vi "1.vi"() -> ()   [LabVIEW 2016]
panel:
  out "Trace Position":dbl[](array[numeric])
  in  "Read Position":bool
  in  "Number of Seconds to Store":dbl=60.0
  in  "Apply X Scale":bool
  in  "Send Handshake":bool=TRUE
  out "DeviceIDs arranged by Type":u8[][](array[numeric])
  out "RoboRIO Net Address":u32
  out "Graph":cluster{sgl[], dbl[]}[](graph)
  in  "Update All Plots":bool
  in  "Reassign IP":bool
  in  "RoboRIO IP Address":string="10.27.67.2"
  in  "Plots":T1={"0"={"DeviceType"=2, "DeviceID"=0, "PropertyID"=1, "Current Value"=0.08333333333333333, "Y-Axis"=0, "Plot Color"=16777215, "Point Color"=16777216}, "0 2"={"DeviceType"=2, "DeviceID"=0, "PropertyID"=1, "Current Value"=50.0, "Y-Axis"=0, "Plot Color"=16777215, "Point Color"=16777216}, "0 3"={"DeviceType"=2, "DeviceID"=0, "PropertyID"=1, "Current Value"=50.0, "Y-Axis"=0, "Plot Color"=16777215, "Point Color"=16777216}, "0 4"={"DeviceType"=2, "DeviceID"=0, "PropertyID"=1, "Current Value"=50.0, "Y-Axis"=0, "Plot Color"=16777215, "Point Color"=16777216}, "0 5"={"DeviceType"=2, "DeviceID"=0, "PropertyID"=1, "Current Value"=50.0, "Y-Axis"=0, "Plot Color"=16777215, "Point Color"=16777216}, "0 6"={"DeviceType"=2, "DeviceID"=0, "PropertyID"=1, "Current Value"=50.0, "Y-Axis"=0, "Plot Color"=16777215, "Point Color"=16777216}, "0 7"={"DeviceType"=2, "DeviceID"=0, "PropertyID"=1, "Current Value"=50.0, "Y-Axis"=0, "Plot Color"=16777215, "Point Color"=16777216}, "0 8"={"DeviceType"=2, "DeviceID"=0, "PropertyID"=1, "Current Value"=50.0, "Y-Axis"=0, "Plot Color"=16777215, "Point Color"=16777216}, "0 9"={"DeviceType"=2, "DeviceID"=0, "PropertyID"=1, "Current Value"=50.0, "Y-Axis"=0, "Plot Color"=16777215, "Point Color"=16777216}, "0 10"={"DeviceType"=2, "DeviceID"=0, "PropertyID"=1, "Current Value"=50.0, "Y-Axis"=0, "Plot Color"=16777215, "Point Color"=16777216}, "0 11"={"DeviceType"=2, "DeviceID"=0, "PropertyID"=1, "Current Value"=50.0, "Y-Axis"=0, "Plot Color"=16777215, "Point Color"=16777216}, "0 12"={"DeviceType"=2, "DeviceID"=0, "PropertyID"=1, "Current Value"=50.0, "Y-Axis"=0, "Plot Color"=16777215, "Point Color"=16777216}, "0 13"={"DeviceType"=2, "DeviceID"=0, "PropertyID"=1, "Current Value"=50.0, "Y-Axis"=0, "Plot Color"=16777215, "Point Color"=16777216}, "0 14"={"DeviceType"=2, "DeviceID"=0, "PropertyID"=1, "Current Value"=50.0, "Y-Axis"=0, "Plot Color"=16777215, "Point Color"=16777216}, "0 15"={"DeviceType"=2, "DeviceID"=0, "PropertyID"=1, "Current Value"=50.0, "Y-Axis"=0, "Plot Color"=16777215, "Point Color"=16777216}, "0 16"={"DeviceType"=2, "DeviceID"=0, "PropertyID"=1, "Current Value"=50.0, "Y-Axis"=0, "Plot Color"=16777215, "Point Color"=16777216}} {"0 16"."DeviceID" items=["0"]; "0 16"."PropertyID" items=["PacketCounter", "Milliseconds Per Packet", "CPU Load"]; "0 16"."DeviceType" items=["Talon", "DIO", "RoboRIO"]; "0 16"."Y-Axis" items=["Red", "Green", "Blue", "Yellow"]; "0 15"."DeviceID" items=["0"]; "0 15"."PropertyID" items=["PacketCounter", "Milliseconds Per Packet", "CPU Load"]; "0 15"."DeviceType" items=["Talon", "DIO", "RoboRIO"]; "0 15"."Y-Axis" items=["Red", "Green", "Blue", "Yellow"]; "0 14"."DeviceID" items=["0"]; "0 14"."PropertyID" items=["PacketCounter", "Milliseconds Per Packet", "CPU Load"]; "0 14"."DeviceType" items=["Talon", "DIO", "RoboRIO"]; "0 14"."Y-Axis" items=["Red", "Green", "Blue", "Yellow"]; "0 13"."DeviceID" items=["0"]; "0 13"."PropertyID" items=["PacketCounter", "Milliseconds Per Packet", "CPU Load"]; "0 13"."DeviceType" items=["Talon", "DIO", "RoboRIO"]; "0 13"."Y-Axis" items=["Red", "Green", "Blue", "Yellow"]; "0 12"."DeviceID" items=["0"]; "0 12"."PropertyID" items=["PacketCounter", "Milliseconds Per Packet", "CPU Load"]; "0 12"."DeviceType" items=["Talon", "DIO", "RoboRIO"]; "0 12"."Y-Axis" items=["Red", "Green", "Blue", "Yellow"]; "0 11"."DeviceID" items=["0"]; "0 11"."PropertyID" items=["PacketCounter", "Milliseconds Per Packet", "CPU Load"]; "0 11"."DeviceType" items=["Talon", "DIO", "RoboRIO"]; "0 11"."Y-Axis" items=["Red", "Green", "Blue", "Yellow"]; "0 10"."DeviceID" items=["0"]; "0 10"."PropertyID" items=["PacketCounter", "Milliseconds Per Packet", "CPU Load"]; "0 10"."DeviceType" items=["Talon", "DIO", "RoboRIO"]; "0 10"."Y-Axis" items=["Red", "Green", "Blue", "Yellow"]; "0 9"."DeviceID" items=["0"]; "0 9"."PropertyID" items=["PacketCounter", "Milliseconds Per Packet", "CPU Load"]; "0 9"."DeviceType" items=["Talon", "DIO", "RoboRIO"]; "0 9"."Y-Axis" items=["Red", "Green", "Blue", "Yellow"]; "0 8"."DeviceID" items=["0"]; "0 8"."PropertyID" items=["PacketCounter", "Milliseconds Per Packet", "CPU Load"]; "0 8"."DeviceType" items=["Talon", "DIO", "RoboRIO"]; "0 8"."Y-Axis" items=["Red", "Green", "Blue", "Yellow"]; "0 7"."DeviceID" items=["0"]; "0 7"."PropertyID" items=["PacketCounter", "Milliseconds Per Packet", "CPU Load"]; "0 7"."DeviceType" items=["Talon", "DIO", "RoboRIO"]; "0 7"."Y-Axis" items=["Red", "Green", "Blue", "Yellow"]; "0 6"."DeviceID" items=["0"]; "0 6"."PropertyID" items=["PacketCounter", "Milliseconds Per Packet", "CPU Load"]; "0 6"."DeviceType" items=["Talon", "DIO", "RoboRIO"]; "0 6"."Y-Axis" items=["Red", "Green", "Blue", "Yellow"]; "0 5"."DeviceID" items=["0"]; "0 5"."PropertyID" items=["PacketCounter", "Milliseconds Per Packet", "CPU Load"]; "0 5"."DeviceType" items=["Talon", "DIO", "RoboRIO"]; "0 5"."Y-Axis" items=["Red", "Green", "Blue", "Yellow"]; "0 4"."DeviceID" items=["0"]; "0 4"."PropertyID" items=["PacketCounter", "Milliseconds Per Packet", "CPU Load"]; "0 4"."DeviceType" items=["Talon", "DIO", "RoboRIO"]; "0 4"."Y-Axis" items=["Red", "Green", "Blue", "Yellow"]; "0 3"."DeviceID" items=["0"]; "0 3"."PropertyID" items=["PacketCounter", "Milliseconds Per Packet", "CPU Load"]; "0 3"."DeviceType" items=["Talon", "DIO", "RoboRIO"]; "0 3"."Y-Axis" items=["Red", "Green", "Blue", "Yellow"]; "0 2"."DeviceID" items=["0"]; "0 2"."PropertyID" items=["PacketCounter", "Milliseconds Per Packet", "CPU Load"]; "0 2"."DeviceType" items=["Talon", "DIO", "RoboRIO"]; "0 2"."Y-Axis" items=["Red", "Green", "Blue", "Yellow"]; "0"."DeviceID" items=["0"]; "0"."PropertyID" items=["PacketCounter", "Milliseconds Per Packet", "CPU Load"]; "0"."DeviceType" items=["Talon", "DIO", "RoboRIO"]; "0"."Y-Axis" items=["Red", "Green", "Blue", "Yellow"]}
  in  "Load Config":bool
  in  "Save Config":bool
  in  "Configuation Path":path
  out "Real Milliseconds per Packet":sgl=50.0
  in  "Apply New Milliseconds":bool
  in  "Milliseconds per Packet":sgl=50.0
  in  "Number of Seconds Visible":dbl=10.0
  in  "Stop Data":bool
  # "Grapher v7.0"
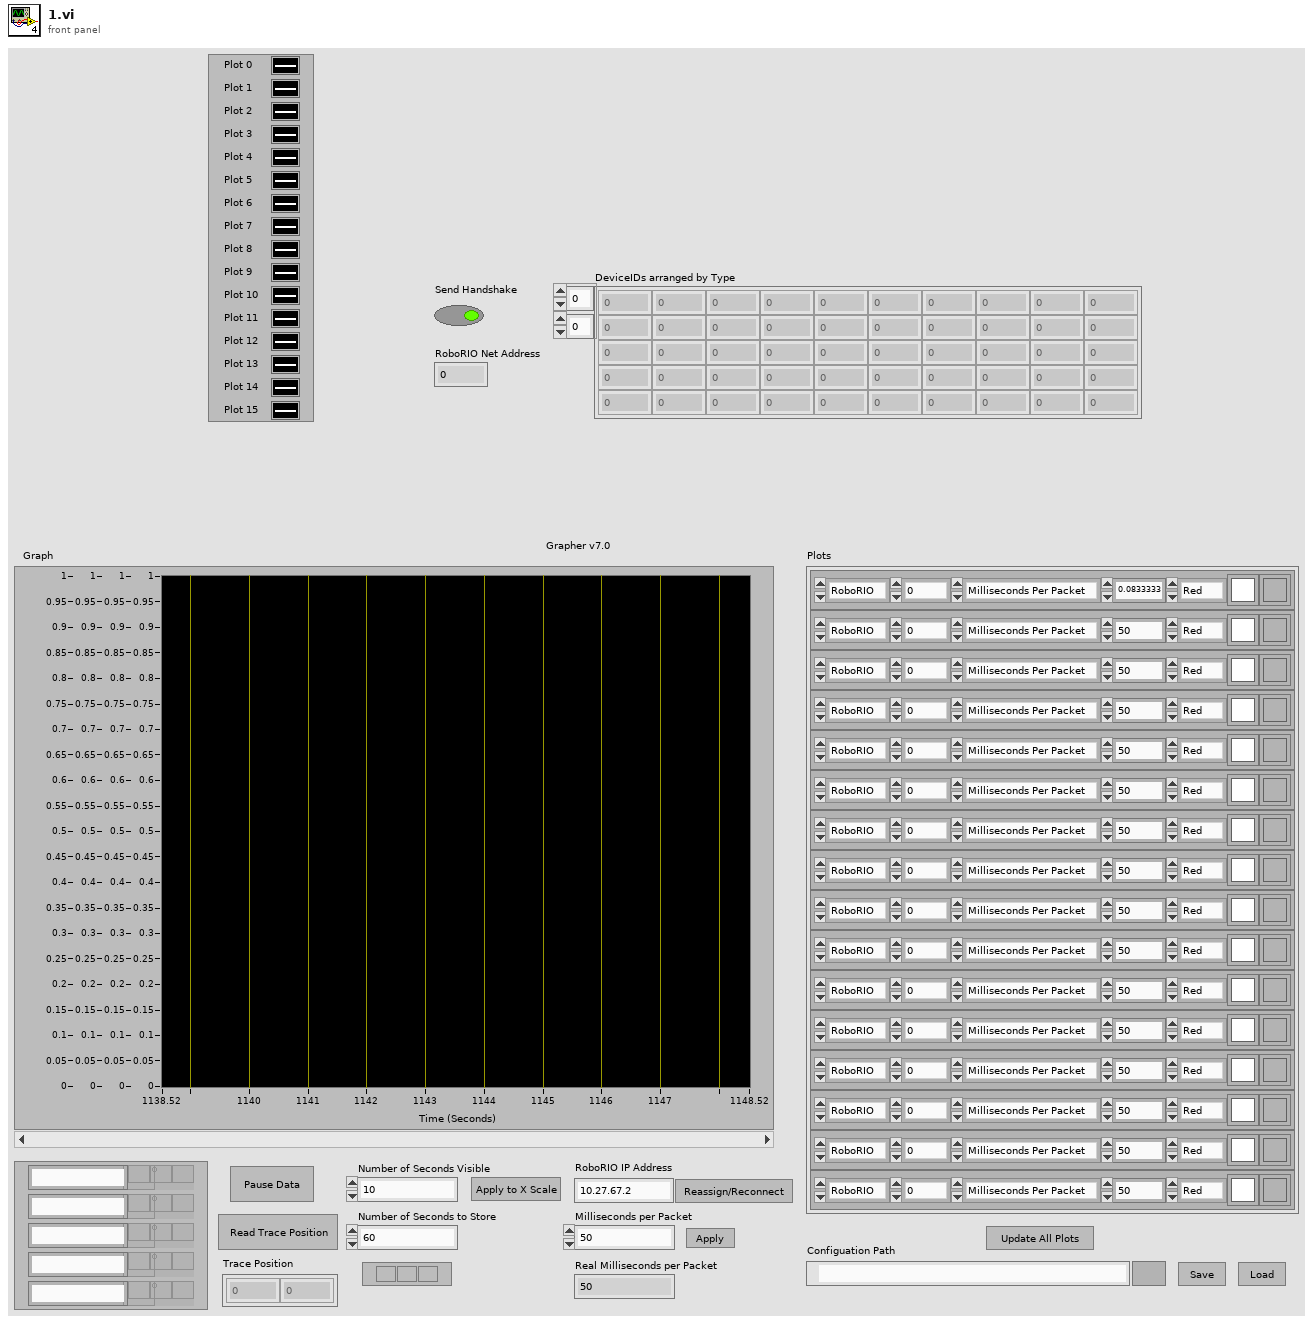
[diagram p1: front panel]
types:
  T1 = cluster{"0":cluster{"DeviceType":u8, "DeviceID":u8, "PropertyID":u8, "Current Value":dbl, "Y-Axis":u16, "Plot Color":u32, "Point Color":u32}, "0 2":cluster{"DeviceType":u8, "DeviceID":u8, "PropertyID":u8, "Current Value":dbl, "Y-Axis":u16, "Plot Color":u32, "Point Color":u32}, "0 3":cluster{"DeviceType":u8, "DeviceID":u8, "PropertyID":u8, "Current Value":dbl, "Y-Axis":u16, "Plot Color":u32, "Point Color":u32}, "0 4":cluster{"DeviceType":u8, "DeviceID":u8, "PropertyID":u8, "Current Value":dbl, "Y-Axis":u16, "Plot Color":u32, "Point Color":u32}, "0 5":cluster{"DeviceType":u8, "DeviceID":u8, "PropertyID":u8, "Current Value":dbl, "Y-Axis":u16, "Plot Color":u32, "Point Color":u32}, "0 6":cluster{"DeviceType":u8, "DeviceID":u8, "PropertyID":u8, "Current Value":dbl, "Y-Axis":u16, "Plot Color":u32, "Point Color":u32}, "0 7":cluster{"DeviceType":u8, "DeviceID":u8, "PropertyID":u8, "Current Value":dbl, "Y-Axis":u16, "Plot Color":u32, "Point Color":u32}, "0 8":cluster{"DeviceType":u8, "DeviceID":u8, "PropertyID":u8, "Current Value":dbl, "Y-Axis":u16, "Plot Color":u32, "Point Color":u32}, "0 9":cluster{"DeviceType":u8, "DeviceID":u8, "PropertyID":u8, "Current Value":dbl, "Y-Axis":u16, "Plot Color":u32, "Point Color":u32}, "0 10":cluster{"DeviceType":u8, "DeviceID":u8, "PropertyID":u8, "Current Value":dbl, "Y-Axis":u16, "Plot Color":u32, "Point Color":u32}, "0 11":cluster{"DeviceType":u8, "DeviceID":u8, "PropertyID":u8, "Current Value":dbl, "Y-Axis":u16, "Plot Color":u32, "Point Color":u32}, "0 12":cluster{"DeviceType":u8, "DeviceID":u8, "PropertyID":u8, "Current Value":dbl, "Y-Axis":u16, "Plot Color":u32, "Point Color":u32}, "0 13":cluster{"DeviceType":u8, "DeviceID":u8, "PropertyID":u8, "Current Value":dbl, "Y-Axis":u16, "Plot Color":u32, "Point Color":u32}, "0 14":cluster{"DeviceType":u8, "DeviceID":u8, "PropertyID":u8, "Current Value":dbl, "Y-Axis":u16, "Plot Color":u32, "Point Color":u32}, "0 15":cluster{"DeviceType":u8, "DeviceID":u8, "PropertyID":u8, "Current Value":dbl, "Y-Axis":u16, "Plot Color":u32, "Point Color":u32}, "0 16":cluster{"DeviceType":u8, "DeviceID":u8, "PropertyID":u8, "Current Value":dbl, "Y-Axis":u16, "Plot Color":u32, "Point Color":u32}}
  T2 = enum8{"DeviceListRequest", "DeviceList", "UpdateSubscription", "SubscriptionData"}
  T3 = enum8{"DeviceListRequest", "DeviceList", "UpdateSubscription", "SubscriptionData", "ChangeUpdateRate"}
  T4 = enum16{"open", "replace", "create", "open or create", "replace or create", "replace or create with confirmation"}
  T5 = cluster{"YScale.Maximum":dbl, "YScale.Minimum":dbl}
  T6 = typedef "LVAnnotationListTypeDef.ctl" = cluster{"Name":string, "Color":u32, "Style":u8, "Point Style":u8, "Name Visible":bool, "Allow Drag":bool, "Annotation Mode":u32, "Plot":i32, "Index":i32, "Position":cluster{"X":dbl, "Y":dbl}, "X Scale":u32, "Y Scale":u32, "Show Arrow":bool, "Lock Name":bool, "Plot Area":i32, "Label Offset":cluster{"X":dbl, "Y":dbl}}[]
  T7 = cluster{"Name":string, "Color":u32, "Style":u8, "Point Style":u8, "Name Visible":bool, "Allow Drag":bool, "Annotation Mode":u32, "Plot":i32, "Index":i32, "Position":cluster{"X":dbl, "Y":dbl}, "X Scale":u32, "Y Scale":u32, "Show Arrow":bool, "Lock Name":bool, "Plot Area":i32, "Label Offset":cluster{"X":dbl, "Y":dbl}}
  T8 = cluster{enum8{"DeviceListRequest", "DeviceList", "UpdateSubscription", "SubscriptionData"}, u8, "unsigned 8bit integer":u8, "unsigned 8bit integer":u8, "unsigned 8bit integer":u8}
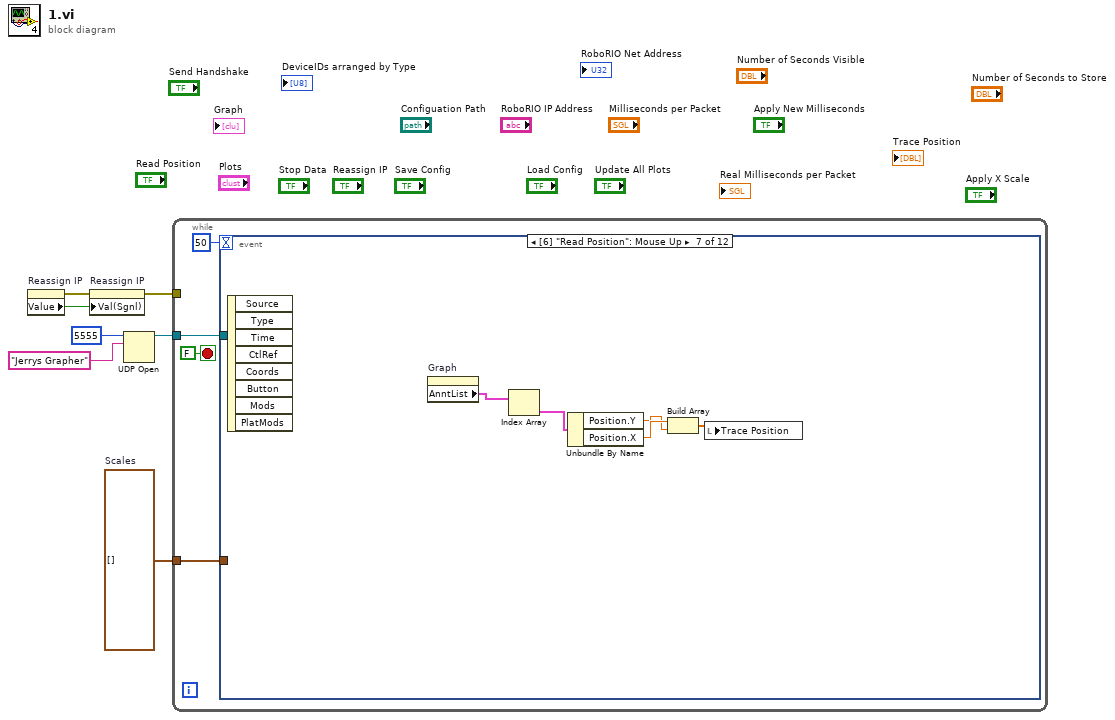
[diagram p0: block diagram]
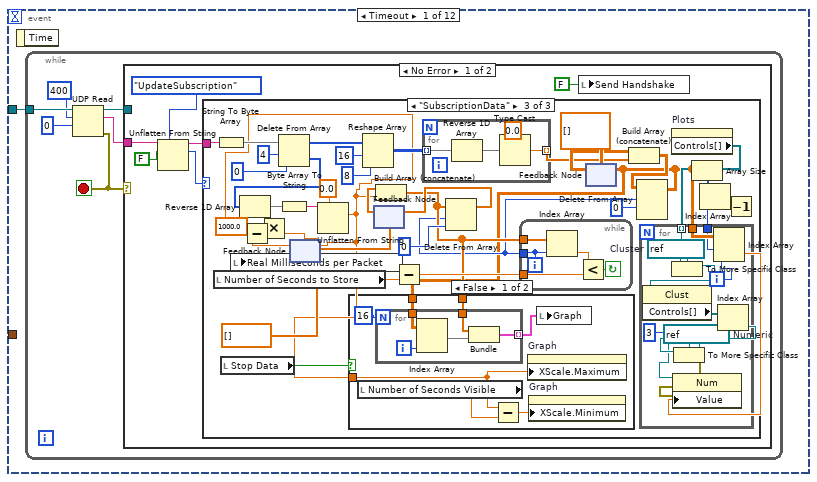
[diagram p2: hidden frame]
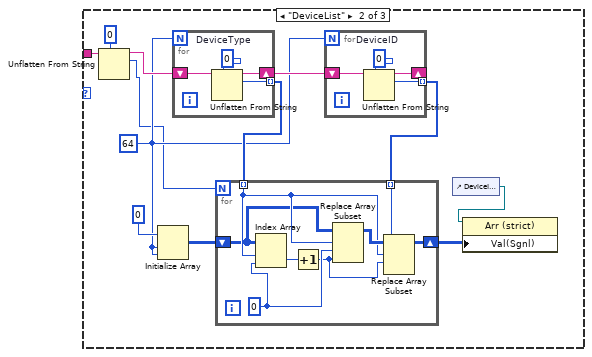
[diagram p4: hidden frame]
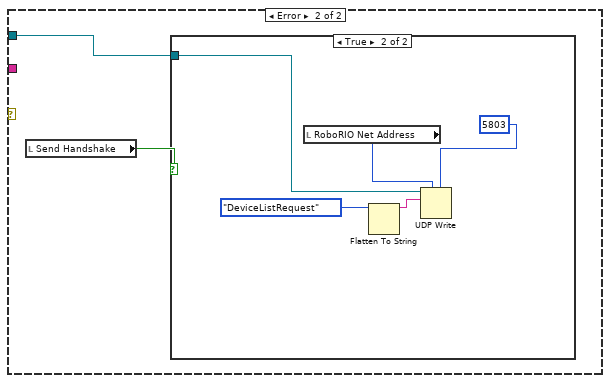
[diagram p6: hidden frame]
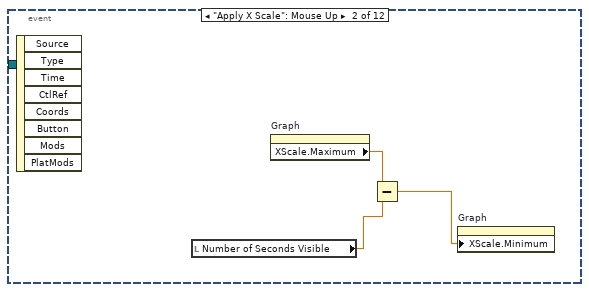
[diagram p8: hidden frame]
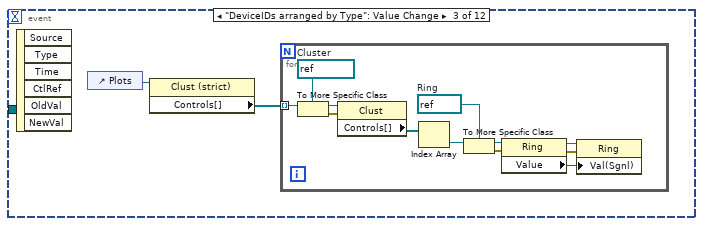
[diagram p9: hidden frame]
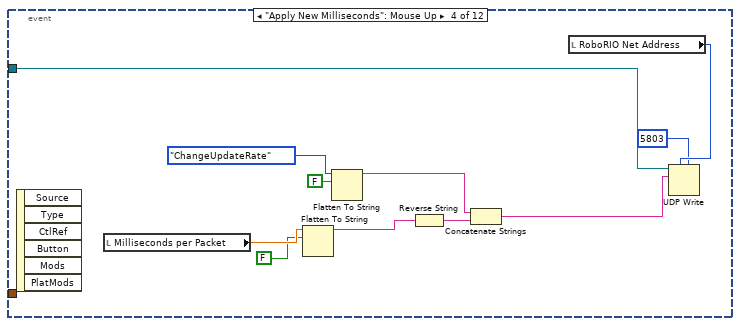
[diagram p10: hidden frame]
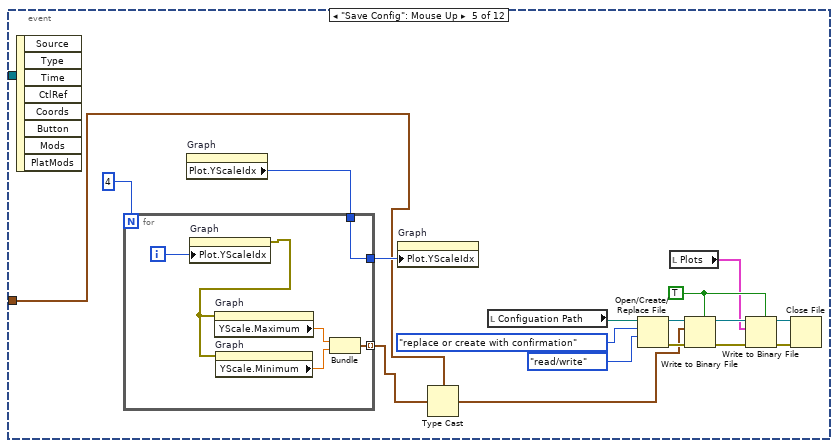
[diagram p11: hidden frame]
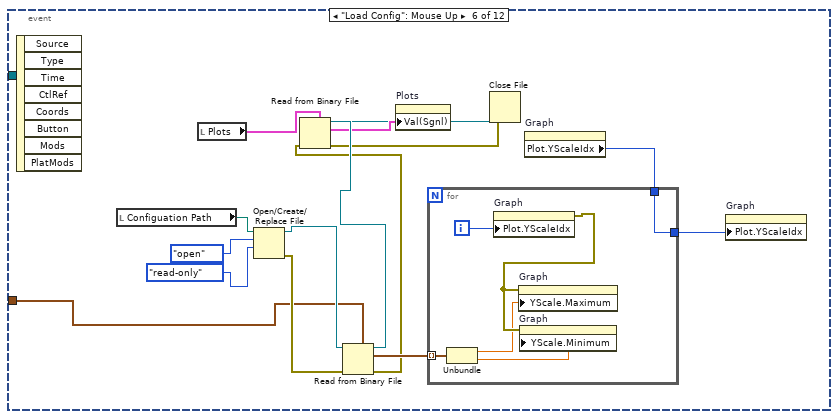
[diagram p12: hidden frame]
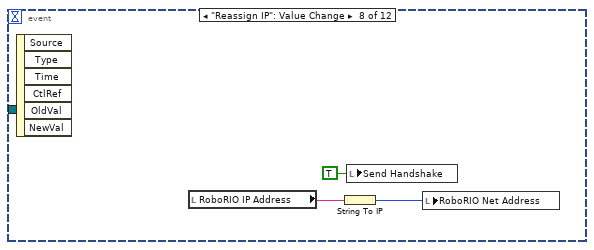
[diagram p13: hidden frame]
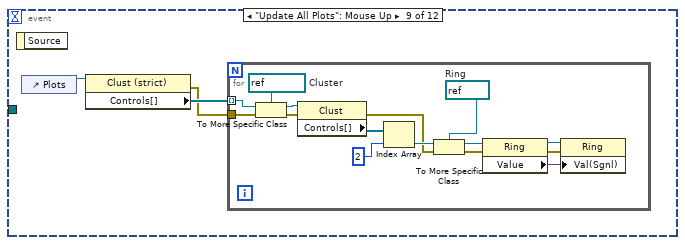
[diagram p14: hidden frame]
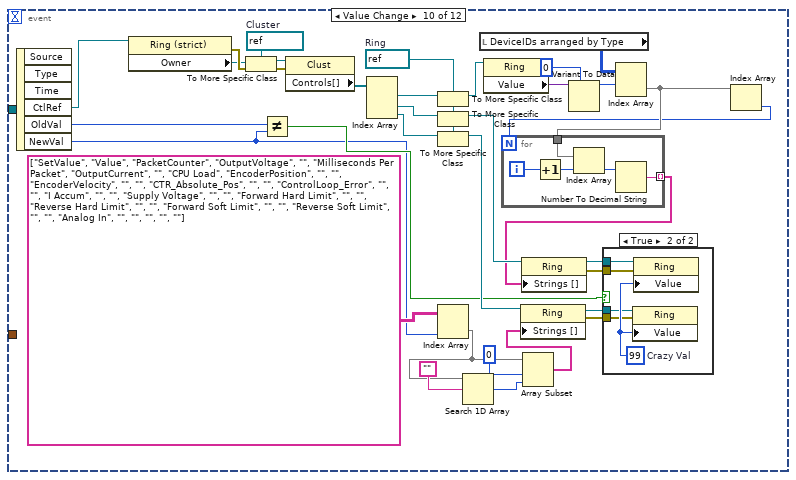
[diagram p15: hidden frame]
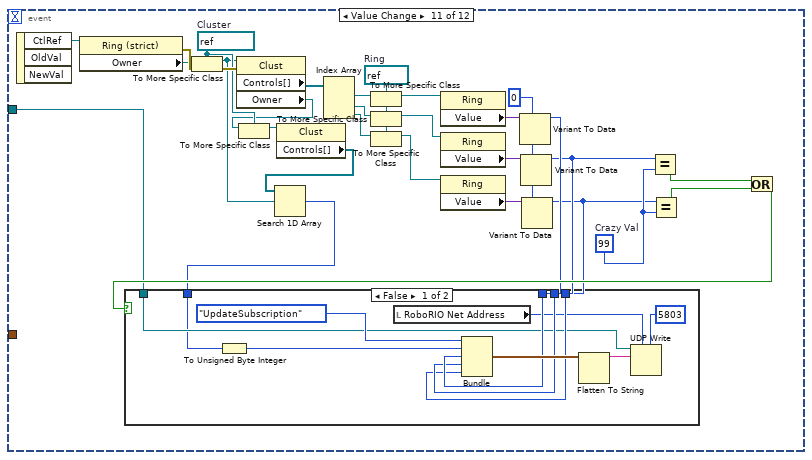
[diagram p17: hidden frame]
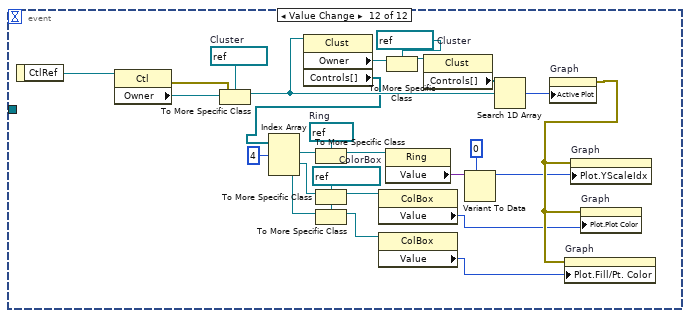
[diagram p19: hidden frame]
diagram:
  w1 = cluster{"Max":dbl, "Min":dbl}[] []  # Scales
  n1 = property on="Reassign IP" class="Bool (strict)"() -> (error out=w6:errorcluster, "Value"=w7:bool)  [unwired: 2 in, 1 out]
  n2 = property on="Reassign IP" class="Bool (strict)"(error in=w6, "Val(Sgnl)"=w7) -> (error out=w5:errorcluster)  [unwired: 1 in, 1 out]
  n3 = UDP Open(10:"Jerrys Grapher" ("service name"), 11:u16 5555 ("port")) -> (port=w4:refnum<k16>)  [unwired: 3 in, 2 out]
  n4 = while {
    tunnel: w5 -> [_]
    tunnel: w4 -> [w9]
    tunnel: w1 -> [w8]
    stop <- FALSE stop-if-true
    n5 = event shown="[6] \"Read Position\": Mouse Up" {
      selector: _ -> [_ _ _ _ _ _ _ _ _ _ _ _]
      dyn-events: _ -> [_ _ _ _ _ _ _ _ _ _ _ _]
      timeout: 50 -> [_ _ _ _ _ _ _ _ _ _ _ _]
      tunnel: w9 -> [w12 _ _ w149 _ _ _ _ _ _ w280 _]
      tunnel: w8 -> [_ _ _ _ w158 w181 _ _ _ _ _ _]
      event Timeout {
        n6 = event-data() -> ()  [unwired: 1 in, 1 out]
        n7 = while {
          tunnel: w12 -> [w18]
          stop <- w13 stop-if-true
          n8 = UDP Read(connection ID=w18, max size (548)=400 ("timeout ms (25000)"), timeout ms (25000)=0) -> (data out=w17:string, error out=w13:errorcluster, 3:w14:refnum<k16>)  [unwired: 1 in, 2 out]
          n9 = case shown="No Error" w13 {
            tunnel: w17 -> [w23 _]
            tunnel: w14 -> [_ w124]
            frame No Error {
              n10 = Unflatten From String(type=T2."UpdateSubscription", binary string=w23, data includes array or string size? (T)=FALSE) -> (rest of the binary string=w20:string, value=w21:T2)  [unwired: 2 in, 1 out]
              n11 = case shown="\"SubscriptionData\"" w21 {
                tunnel: w20 -> [_ w35 w85]
                frame "DeviceListRequest", Default {
                }
                frame "DeviceList" {
                  w26 = 64 ("JERRYSGRAPHER_MAX_NUMBER_OF_DEVICES")
                  n12 = Unflatten From String(type=u8 0 ("Number of Devices"), binary string=w35) -> (rest of the binary string=w34:string, value=w25:u8)  [unwired: 3 in, 1 out]
                  n13 = Initialize Array(u8 0, w26, w26) -> (w31:u8[][])
                  n14 = for {
                    N: w26 -> [_]
                    shift-right: [w49] -> w33
                    shift-left: w34 -> [w51]
                    tunnel: [w50] -> w30 mode=indexing
                    w52 = u8 0  # DeviceType
                    n15 = Unflatten From String(type=w52, binary string=w51) -> (rest of the binary string=w49:string, value=w50:u8)  [unwired: 3 in, 1 out]
                  }
                  n16 = for {
                    N: w26 -> [_]
                    shift-right: [w45] -> _
                    shift-left: w33 -> [w47]
                    tunnel: [w46] -> w29 mode=indexing
                    w48 = u8 0  # DeviceID
                    n17 = Unflatten From String(type=w48, binary string=w47) -> (rest of the binary string=w45:string, value=w46:u8)  [unwired: 3 in, 1 out]
                  }
                  n18 = for {
                    N: w25 -> [_]
                    tunnel: w30 -> [w42] mode=indexing
                    tunnel: w29 -> [w38] mode=indexing
                    shift-right: [w44] -> w28
                    shift-left: w31 -> [w40]
                    w41 = 0 ("disabled index (col)")
                    n19 = Index Array(array=w40, index (row)=w42, index (col)=w41) -> (element=w39:u8)
                    n20 = Increment(x=w39) -> (x+1=w37:u8)
                    n21 = Replace Array Subset(array=w40, new element=w37, index (row)=w42, index (col)=w41) -> (w43:u8[][])
                    n22 = Replace Array Subset(array=w43, new element=w38, index (row)=w42, index (col)=w37) -> (w44:u8[][])
                  }
                  n23 = control-ref of="DeviceIDs arranged by Type"() -> (w27:refnum<vi>)
                  n24 = property class="Arr (strict)"(reference=w27, "Val(Sgnl)"=w28) -> ()  [unwired: 1 in, 2 out]
                }
                frame "SubscriptionData" {
                  n25 = local read "Number of Seconds to Store"() -> (w70:dbl)
                  n26 = String To Byte Array(string=w85) -> (unsigned byte array=w86:u8[])
                  n27 = local read "Stop Data"() -> (w72:bool)
                  n28 = Delete From Array(array=w86, length=4, index=0) -> (deleted portion=w73:u8[], array with subset deleted=w80:u8[])
                  n29 = Reverse 1D Array(array=w73) -> (reversed array=w83:u8[])
                  n30 = Byte Array To String(unsigned byte array=w83) -> (string=w82:string)
                  n31 = feedback #1() -> (w56:sgl)  [unwired: 1 in]
                  n32 = Unflatten From String(type=sgl 0.0, binary string=w82) -> (value=w57:sgl)  [unwired: 3 in, 2 out]
                  n33 = Subtract(x=w57, y=w56) -> (x-y=w55:sgl)
                  n34 = Multiply(x=sgl 1000.0, y=w55) -> (x*y=w54:sgl)
                  n35 = local write "Real Milliseconds per Packet"(w54) -> ()
                  n36 = feedback-in #1(w57) -> ()
                  n37 = Reshape Array(w80, 16 ("dimension size"), 8 ("dimension size")) -> (w81:u8[][])
                  n38 = feedback #2(sgl[] []) -> (w77:sgl[])
                  n39 = Build Array (concatenate)(w77, w57) -> (w64:sgl[])
                  n40 = Subtract(x=w57, y=w70) -> (x-y=w69:dbl)
                  n41 = for {
                    tunnel: [w122] -> w74 mode=indexing
                    tunnel: w81 -> [w120] mode=indexing
                    n42 = Reverse 1D Array(array=w120) -> (reversed array=w119:u8[])
                    n43 = Type Cast(type=0.0, x=w119) -> (*(type *) &x=w122:dbl)
                  }
                  n44 = while {
                    tunnel: w69 -> [w104]
                    tunnel: w64 -> [w103]
                    tunnel: [w102] -> w63
                    i -> [w102]
                    stop <- w106 continue-if-true
                    n45 = Index Array(array=w103, index=w102) -> (element=w105:sgl)
                    n46 = Less?(x=w105, y=w104) -> (x < y?=w106:bool)
                  }
                  n47 = Delete From Array(array=w64, length=w63, index=0) -> (array with subset deleted=w67:sgl[])  [unwired: 1 out]
                  n48 = feedback-in #2(w67) -> ()
                  n49 = feedback #3(dbl[][] []) -> (w75:dbl[][])
                  n50 = Build Array (concatenate)(w75, w74) -> (w66:dbl[][])
                  n51 = Delete From Array(array=w66, length=w63, index (row)=0) -> (array with subset deleted=w61:dbl[][])  [unwired: 1 in, 1 out]
                  n52 = case shown="False" w72 {
                    tunnel: w57 -> [w113 _]
                    tunnel: w61 -> [w109 _]
                    tunnel: w64 -> [w108 _]
                    frame False {
                      n53 = local read "Number of Seconds Visible"() -> (w112:dbl)
                      n54 = for {
                        N: 16 -> [_]
                        tunnel: [w118] -> w107 mode=indexing
                        tunnel: w109 -> [w115]
                        tunnel: w108 -> [w114]
                        i -> [w117]
                        n55 = Index Array(array=w115, index (col)=w117) -> (element=w116:dbl[])  [unwired: 1 in]
                        n56 = Bundle(w114, w116) -> (w118:cluster{sgl[], dbl[]})  [unwired: 1 in]
                      }
                      n57 = Subtract(x=w113, y=w112) -> (x-y=w111:dbl)
                      n58 = property on="Graph" class="XYGraph (strict)"("XScale.Maximum"=w113) -> ()  [unwired: 2 in, 2 out]
                      n59 = property on="Graph" class="XYGraph (strict)"("XScale.Minimum"=w111) -> ()  [unwired: 2 in, 2 out]
                      n60 = local write "Graph"(w107) -> ()
                    }
                    frame True {
                    }
                  }
                  n61 = feedback-in #3(w61) -> ()
                  n62 = property on="Plots" class="Clust (strict)"() -> ("Controls[]"=w62:refnum<vi>[])  [unwired: 2 in, 2 out]
                  n63 = Array Size(array=w61) -> (size(s)=w60:i32[])
                  n64 = Index Array(array=w60) -> (element=w59:i32)  [unwired: 1 in]
                  n65 = Decrement(x=w59) -> (x-1=w58:i32)
                  n66 = for {
                    tunnel: w62 -> [w101] mode=indexing
                    tunnel: w61 -> [w92]
                    tunnel: w58 -> [w90]
                    i -> [w89]
                    w96 = refnum<vi> refnum  # Numeric
                    w100 = refnum<vi> refnum  # Cluster
                    n67 = To More Specific Class(target class=w100, reference=w101) -> (specific class reference=w99:refnum<vi>)  [unwired: 1 in, 1 out]
                    n68 = property class="Clust"(reference=w99) -> ("Controls[]"=w98:refnum<vi>[])  [unwired: 1 in, 2 out]
                    n69 = Index Array(array=w92, index (row)=w90, index (col)=w89) -> (element=w91:dbl)
                    n70 = Index Array(array=w98, index=3) -> (element=w95:refnum<vi>)
                    n71 = To More Specific Class(target class=w96, reference=w95) -> (specific class reference=w94:refnum<vi>, error out=w93:errorcluster)  [unwired: 1 in]
                    n72 = property class="Num"(reference=w94, error in=w93, "Value"=w91) -> ()  [unwired: 2 out]
                  }
                }
              }
              n73 = local write "Send Handshake"(FALSE ("Send Handshake")) -> ()
            }
            frame Error {
              n74 = local read "Send Handshake"() -> (w123:bool)
              n75 = case shown="True" w123 {
                tunnel: w124 -> [_ w127]
                frame False {
                }
                frame True {
                  n76 = local read "RoboRIO Net Address"() -> (w126:u32)
                  n77 = Flatten To String(anything=T2."DeviceListRequest") -> (data string=w128:string)  [unwired: 3 in, 2 out]
                  n78 = UDP Write(address=w126, port or service name=u16 5803 ("port"), connection ID=w127, data in=w128) -> ()  [unwired: 2 in, 2 out]
                }
              }
            }
          }
        }
      }
      event "Apply X Scale": Mouse Up {
        n79 = event-data() -> ()  [unwired: 1 in, 8 out]
        n80 = local read "Number of Seconds Visible"() -> (w131:dbl)
        n81 = property on="Graph" class="XYGraph (strict)"() -> ("XScale.Maximum"=w132:dbl)  [unwired: 2 in, 2 out]
        n82 = Subtract(x=w132, y=w131) -> (x-y=w130:dbl)
        n83 = property on="Graph" class="XYGraph (strict)"("XScale.Minimum"=w130) -> ()  [unwired: 2 in, 2 out]
      }
      event "DeviceIDs arranged by Type": Value Change {
        n84 = event-data() -> ()  [unwired: 1 in, 6 out]
        n85 = control-ref of="Plots"() -> (w134:refnum<vi>)
        n86 = property class="Clust (strict)"(reference=w134) -> ("Controls[]"=w133:refnum<vi>[])  [unwired: 1 in, 2 out]
        n87 = for {
          tunnel: w133 -> [w144] mode=indexing
          w140 = refnum<vi> refnum  # Ring
          w143 = refnum<vi> refnum  # Cluster
          n88 = To More Specific Class(target class=w143, reference=w144) -> (specific class reference=w145:refnum<vi>, error out=w146:errorcluster)  [unwired: 1 in]
          n89 = property class="Clust"(reference=w145, error in=w146) -> ("Controls[]"=w142:refnum<vi>[])  [unwired: 2 out]
          n90 = Index Array(array=w142) -> (element=w141:refnum<vi>)  [unwired: 1 in]
          n91 = To More Specific Class(target class=w140, reference=w141) -> (specific class reference=w139:refnum<vi>, error out=w138:errorcluster)  [unwired: 1 in]
          n92 = property class="Ring"(reference=w139, error in=w138) -> (reference out=w137:refnum<vi>, error out=w136:errorcluster, "Value"=w135:variant)
          n93 = property class="Ring"(reference=w137, error in=w136, "Val(Sgnl)"=w135) -> ()  [unwired: 2 out]
        }
      }
      event "Apply New Milliseconds": Mouse Up {
        n94 = event-data() -> ()  [unwired: 1 in, 6 out]
        n95 = local read "Milliseconds per Packet"() -> (w152:sgl)
        n96 = Flatten To String(anything=w152, prepend array or string size? (T)=FALSE) -> (data string=w154:string)  [unwired: 2 in, 2 out]
        n97 = Flatten To String(anything=T3."ChangeUpdateRate", prepend array or string size? (T)=FALSE) -> (data string=w153:string)  [unwired: 2 in, 2 out]
        n98 = Reverse String(1:w154) -> (0:w157:string)
        n99 = Concatenate Strings(w153, w157) -> (w156:string)
        n100 = local read "RoboRIO Net Address"() -> (w148:u32)
        n101 = UDP Write(address=w148, port or service name=u16 5803, connection ID=w149, data in=w156) -> ()  [unwired: 2 in, 2 out]
      }
      event "Save Config": Mouse Up {
        w171 = TRUE ("prepend array or string size? (T)")
        n102 = event-data() -> ()  [unwired: 1 in, 8 out]
        n103 = property on="Graph" class="XYGraph (strict)"() -> ("Plot.YScaleIdx"=w163:u32)  [unwired: 2 in, 2 out]
        n104 = for {
          N: 4 -> [_]
          tunnel: [w176] -> w164
          tunnel: w163 -> [w176]
          tunnel: [w175] -> w160 mode=indexing
          i -> [w180]
          n105 = property on="Graph" class="XYGraph (strict)"("Plot.YScaleIdx"=w180) -> (error out=w179:errorcluster)  [unwired: 2 in, 1 out]
          n106 = property on="Graph" class="XYGraph (strict)"(error in=w179) -> ("YScale.Maximum"=w178:dbl)  [unwired: 1 in, 2 out]
          n107 = property on="Graph" class="XYGraph (strict)"(error in=w179) -> ("YScale.Minimum"=w177:dbl)  [unwired: 1 in, 2 out]
          n108 = Bundle("YScale.Maximum"=w178, "YScale.Minimum"=w177) -> (w175:T5)  [unwired: 1 in]
        }
        n109 = property on="Graph" class="XYGraph (strict)"("Plot.YScaleIdx"=w164) -> ()  [unwired: 2 in, 2 out]
        n110 = Type Cast(type=w158, x=w160) -> (*(type *) &x=w159:cluster{"Max":dbl, "Min":dbl}[])
        n111 = local read "Configuation Path"() -> (w168:path)
        n112 = Open/Create/Replace File(file path (use dialog)=w168, operation (0:open)=T4."replace or create with confirmation", access (0:read/write)=enum16{"read/write", "read-only", "write-only"}."read/write") -> (refnum out=w170:refnum<file>, error out=w172:errorcluster)  [unwired: 3 in, 1 out]
        n113 = local read "Plots"() -> (w162:T1)
        n114 = Write to Binary File(file (use dialog)=w170, data=w159, error in=w172, 5:w171) -> (refnum out=w169:refnum<file>, error out=w173:errorcluster)  [unwired: 2 in, 1 out]
        n115 = Write to Binary File(file (use dialog)=w169, data=w162, error in=w173, 5:w171) -> (refnum out=w161:refnum<file>, error out=w174:errorcluster)  [unwired: 2 in, 1 out]
        n116 = Close File(refnum=w161, error in=w174) -> ()  [unwired: 2 out]
      }
      event "Load Config": Mouse Up {
        n117 = event-data() -> ()  [unwired: 1 in, 8 out]
        n118 = local read "Configuation Path"() -> (w195:path)
        n119 = local read "Plots"() -> (w187:T1)
        n120 = Open/Create/Replace File(file path (use dialog)=w195, operation (0:open)=T4."open", access (0:read/write)=enum16{"read/write", "read-only", "write-only"}."read-only") -> (refnum out=w192:refnum<file>, error out=w185:errorcluster)  [unwired: 3 in, 1 out]
        n121 = Read from Binary File(5:w181, 8:w185, 11:w192) -> (0:w184:errorcluster, 2:w189:cluster{"Max":dbl, "Min":dbl}[], 3:w188:refnum<file>)  [unwired: 3 in, 1 out]
        n122 = Read from Binary File(5:w187, 8:w184, 11:w188) -> (0:w183:errorcluster, 2:w186:T1, 3:w182:refnum<file>)  [unwired: 3 in, 1 out]
        n123 = property on="Plots" class="Clust (strict)"("Val(Sgnl)"=w186) -> ()  [unwired: 2 in, 2 out]
        n124 = Close File(refnum=w182, error in=w183) -> ()  [unwired: 2 out]
        n125 = property on="Graph" class="XYGraph (strict)"() -> ("Plot.YScaleIdx"=w191:u32)  [unwired: 2 in, 2 out]
        n126 = for {
          tunnel: [w199] -> w190
          tunnel: w191 -> [w199]
          tunnel: w189 -> [w198] mode=indexing
          i -> [w201]
          n127 = Unbundle(w198) -> ("Max"=w197:dbl, "Min"=w196:dbl)
          n128 = property on="Graph" class="XYGraph (strict)"("Plot.YScaleIdx"=w201) -> (error out=w200:errorcluster)  [unwired: 2 in, 1 out]
          n129 = property on="Graph" class="XYGraph (strict)"(error in=w200, "YScale.Maximum"=w197) -> ()  [unwired: 1 in, 2 out]
          n130 = property on="Graph" class="XYGraph (strict)"(error in=w200, "YScale.Minimum"=w196) -> ()  [unwired: 1 in, 2 out]
        }
        n131 = property on="Graph" class="XYGraph (strict)"("Plot.YScaleIdx"=w190) -> ()  [unwired: 2 in, 2 out]
      }
      event "Read Position": Mouse Up {
        n132 = event-data() -> ()  [unwired: 1 in, 8 out]
        n133 = property on="Graph" class="XYGraph (strict)"() -> ("AnntList"=w206:T6)  [unwired: 2 in, 2 out]
        n134 = Index Array(array=w206) -> (element=w205:T7)  [unwired: 1 in]
        n135 = Unbundle By Name(w205) -> ("Position.Y"=w203:dbl, "Position.X"=w204:dbl)
        n136 = Build Array(w204, w203) -> (w202:dbl[])
        n137 = local write "Trace Position"(w202) -> ()
      }
      event "Reassign IP": Value Change {
        n138 = event-data() -> ()  [unwired: 1 in, 6 out]
        n139 = local read "RoboRIO IP Address"() -> (w209:string)
        n140 = String To IP(1:w209) -> (0:w208:u32)
        n141 = local write "Send Handshake"(TRUE ("Send Handshake")) -> ()
        n142 = local write "RoboRIO Net Address"(w208) -> ()
      }
      event "Update All Plots": Mouse Up {
        n143 = event-data() -> ()  [unwired: 1 in, 1 out]
        n144 = control-ref of="Plots"() -> (w212:refnum<vi>)
        n145 = property class="Clust (strict)"(reference=w212) -> (error out=w210:errorcluster, "Controls[]"=w211:refnum<vi>[])  [unwired: 1 in, 1 out]
        n146 = for {
          tunnel: w211 -> [w226] mode=indexing
          tunnel: w210 -> [w223]
          w219 = refnum<vi> refnum  # Ring
          w227 = refnum<vi> refnum  # Cluster
          n147 = To More Specific Class(target class=w227, reference=w226, error in=w223) -> (specific class reference=w225:refnum<vi>, error out=w224:errorcluster)
          n148 = property class="Clust"(reference=w225, error in=w224) -> (error out=w216:errorcluster, "Controls[]"=w222:refnum<vi>[])  [unwired: 1 out]
          n149 = Index Array(array=w222, index=2) -> (element=w220:refnum<vi>)
          n150 = To More Specific Class(target class=w219, reference=w220, error in=w216) -> (specific class reference=w218:refnum<vi>, error out=w217:errorcluster)
          n151 = property class="Ring"(reference=w218, error in=w217) -> (reference out=w215:refnum<vi>, error out=w214:errorcluster, "Value"=w213:variant)
          n152 = property class="Ring"(reference=w215, error in=w214, "Val(Sgnl)"=w213) -> ()  [unwired: 2 out]
        }
      }
      event "Plots.0.DeviceType", "Plots.0 2.DeviceType", "Plots.0 3.DeviceType", "Plots.0 4.DeviceType", "Plots.0 5.DeviceType", "Plots.0 6.DeviceType", "Plots.0 7.DeviceType", "Plots.0 8.DeviceType", "Plots.0 9.DeviceType", "Plots.0 10.DeviceType", "Plots.0 11.DeviceType", "Plots.0 12.DeviceType", "Plots.0 13.DeviceType", "Plots.0 14.DeviceType", "Plots.0 15.DeviceType", "Plots.0 16.DeviceType": Value Change {
        w251 = refnum<vi> refnum  # Ring
        w256 = refnum<vi> refnum  # Cluster
        n153 = event-data() -> ("CtlRef"=w253:refnum<vi>, "OldVal"=w229:u8, "NewVal"=w228:u8)  [unwired: 1 in, 3 out]
        n154 = property class="Ring (strict)"(reference=w253) -> (error out=w255:errorcluster, "Owner"=w254:refnum<vi>)  [unwired: 1 in, 1 out]
        n155 = To More Specific Class(target class=w256, reference=w254, error in=w255) -> (specific class reference=w257:refnum<vi>, error out=w258:errorcluster)
        n156 = Not Equal?(x=w229, y=w228) -> (x != y?=w230:bool)
        n157 = property class="Clust"(reference=w257, error in=w258) -> ("Controls[]"=w259:refnum<vi>[])  [unwired: 2 out]
        n158 = Index Array(array=w259) -> (element #1=w260:refnum<vi>, element #2=w261:refnum<vi>, element #3=w252:refnum<vi>)  [unwired: 3 in]
        n159 = To More Specific Class(target class=w251, reference=w260) -> (specific class reference=w249:refnum<vi>)  [unwired: 1 in, 1 out]
        n160 = To More Specific Class(target class=w251, reference=w261) -> (specific class reference=w242:refnum<vi>)  [unwired: 1 in, 1 out]
        n161 = To More Specific Class(target class=w251, reference=w252) -> (specific class reference=w250:refnum<vi>)  [unwired: 1 in, 1 out]
        n162 = Index Array(array=string[][] [["SetValue", "Value", "PacketCounter"], ["OutputVoltage", "", "Milliseconds Per Packet"], ["OutputCurrent", "", "CPU Load"], ["EncoderPosition", "", ""], ["EncoderVelocity", "", ""], ["CTR_Absolute_Pos", "", ""], ["ControlLoop_Error", "", ""], ["I Accum", "", ""], ["Supply Voltage", "", ""], ["Forward Hard Limit", "", ""], ["Reverse Hard Limit", "", ""], ["Forward Soft Limit", "", ""], ["Reverse Soft Limit", "", ""], ["Analog In", "", ""], ["", "", ""]], index (col)=w228) -> (element=w237:string[])  [unwired: 1 in]
        n163 = Search 1D Array(1D array=w237, element="") -> (index of element=w238:i32)  [unwired: 1 in]
        n164 = local read "DeviceIDs arranged by Type"() -> (w246:u8[][])
        n165 = property class="Ring"(reference=w249) -> ("Value"=w248:variant)  [unwired: 1 in, 2 out]
        n166 = Array Subset(array=w237, index=0, length=w238) -> (w236:string[])
        n167 = property class="Ring"(reference=w250, "Strings []"=w236) -> (reference out=w232:refnum<vi>, error out=w231:errorcluster)  [unwired: 1 in]
        n168 = Variant To Data(type=u8 0 ("DeviceType"), Variant=w248) -> (data=w245:u8)  [unwired: 1 in, 1 out]
        n169 = Index Array(array=w246, index (row)=w245) -> (element=w244:u8[])  [unwired: 1 in]
        n170 = Index Array(array=w244) -> (element=w243:u8)  [unwired: 1 in]
        n171 = for {
          N: w243 -> [_]
          tunnel: w244 -> [w271]
          tunnel: [w267] -> w241 mode=indexing
          i -> [w270]
          n172 = Increment(x=w270) -> (x+1=w269:i32)
          n173 = Index Array(array=w271, index=w269) -> (element=w268:u8)
          n174 = Number To Decimal String(number=w268) -> (decimal integer string=w267:string)  [unwired: 1 in]
        }
        n175 = property class="Ring"(reference=w242, "Strings []"=w241) -> (reference out=w234:refnum<vi>, error out=w233:errorcluster)  [unwired: 1 in]
        n176 = case shown="True" w230 {
          tunnel: w234 -> [_ w266]
          tunnel: w233 -> [_ w265]
          tunnel: w232 -> [_ w263]
          tunnel: w231 -> [_ w262]
          frame False {
          }
          frame True {
            w264 = 99  # Crazy Val
            n177 = property class="Ring"(reference=w263, error in=w262, "Value"=w264) -> ()  [unwired: 2 out]
            n178 = property class="Ring"(reference=w266, error in=w265, "Value"=w264) -> ()  [unwired: 2 out]
          }
        }
      }
      event "Plots.0.DeviceID", "Plots.0.PropertyID", "Plots.0 2.DeviceID", "Plots.0 2.PropertyID", "Plots.0 3.DeviceID", "Plots.0 3.PropertyID", "Plots.0 4.DeviceID", "Plots.0 4.PropertyID", "Plots.0 5.DeviceID", "Plots.0 5.PropertyID", "Plots.0 6.DeviceID", "Plots.0 6.PropertyID", "Plots.0 7.DeviceID", "Plots.0 7.PropertyID", "Plots.0 8.DeviceID", "Plots.0 8.PropertyID", "Plots.0 9.DeviceID", "Plots.0 9.PropertyID", "Plots.0 10.DeviceID", "Plots.0 10.PropertyID", "Plots.0 11.DeviceID", "Plots.0 11.PropertyID", "Plots.0 12.DeviceID", "Plots.0 12.PropertyID", "Plots.0 13.DeviceID", "Plots.0 13.PropertyID", "Plots.0 14.DeviceID", "Plots.0 14.PropertyID", "Plots.0 15.DeviceID", "Plots.0 15.PropertyID", "Plots.0 16.DeviceID", "Plots.0 16.PropertyID": Value Change {
        w287 = 99  # Crazy Val
        w288 = u8 0 ("unsigned 8bit integer")
        w295 = refnum<vi> refnum  # Ring
        w277 = refnum<vi> refnum  # Cluster
        n179 = event-data() -> ("CtlRef"=w278:refnum<vi>)  [unwired: 1 in, 2 out]
        n180 = property class="Ring (strict)"(reference=w278) -> (error out=w298:errorcluster, "Owner"=w297:refnum<vi>)  [unwired: 1 in, 1 out]
        n181 = To More Specific Class(target class=w277, reference=w297, error in=w298) -> (specific class reference=w273:refnum<vi>, error out=w299:errorcluster)
        n182 = property class="Clust"(reference=w273, error in=w299) -> ("Controls[]"=w279:refnum<vi>[], "Owner"=w276:refnum<vi>)  [unwired: 2 out]
        n183 = To More Specific Class(target class=w277, reference=w276) -> (specific class reference=w275:refnum<vi>)  [unwired: 1 in, 1 out]
        n184 = property class="Clust"(reference=w275) -> ("Controls[]"=w274:refnum<vi>[])  [unwired: 1 in, 2 out]
        n185 = Search 1D Array(1D array=w274, element=w273) -> (index of element=w272:i32)  [unwired: 1 in]
        n186 = Index Array(array=w279) -> (element #1=w300:refnum<vi>, element #2=w301:refnum<vi>, element #3=w296:refnum<vi>)  [unwired: 3 in]
        n187 = To More Specific Class(target class=w295, reference=w300) -> (specific class reference=w294:refnum<vi>)  [unwired: 1 in, 1 out]
        n188 = To More Specific Class(target class=w295, reference=w301) -> (specific class reference=w293:refnum<vi>)  [unwired: 1 in, 1 out]
        n189 = To More Specific Class(target class=w295, reference=w296) -> (specific class reference=w292:refnum<vi>)  [unwired: 1 in, 1 out]
        n190 = property class="Ring"(reference=w294) -> ("Value"=w289:variant)  [unwired: 1 in, 2 out]
        n191 = property class="Ring"(reference=w293) -> ("Value"=w290:variant)  [unwired: 1 in, 2 out]
        n192 = property class="Ring"(reference=w292) -> ("Value"=w291:variant)  [unwired: 1 in, 2 out]
        n193 = Variant To Data(type=w288, Variant=w289) -> (data=w283:u8)  [unwired: 1 in, 1 out]
        n194 = Variant To Data(type=w288, Variant=w290) -> (data=w282:u8)  [unwired: 1 in, 1 out]
        n195 = Variant To Data(type=w288, Variant=w291) -> (data=w281:u8)  [unwired: 1 in, 1 out]
        n196 = Equal?(x=w282, y=w287) -> (x = y?=w285:bool)
        n197 = Equal?(x=w281, y=w287) -> (x = y?=w286:bool)
        n198 = Or(x=w285, y=w286) -> (x .or. y?=w284:bool)
        n199 = case shown="False" w284 {
          tunnel: w283 -> [w308 _]
          tunnel: w282 -> [w307 _]
          tunnel: w281 -> [w306 _]
          tunnel: w280 -> [w305 _]
          tunnel: w272 -> [w302 _]
          frame False {
            n200 = To Unsigned Byte Integer(number=w302) -> (unsigned 8bit integer=w309:u8)
            n201 = local read "RoboRIO Net Address"() -> (w304:u32)
            n202 = Bundle(T2."UpdateSubscription", w309, "unsigned 8bit integer"=w308, "unsigned 8bit integer"=w307, "unsigned 8bit integer"=w306) -> (w311:T8)  [unwired: 1 in]
            n203 = Flatten To String(anything=w311) -> (data string=w312:string)  [unwired: 3 in, 2 out]
            n204 = UDP Write(address=w304, port or service name=u16 5803, connection ID=w305, data in=w312) -> ()  [unwired: 2 in, 2 out]
          }
          frame True {
          }
        }
      }
      event "Plots.0.Y-Axis", "Plots.0 2.Y-Axis", "Plots.0 3.Y-Axis", "Plots.0 4.Y-Axis", "Plots.0 5.Y-Axis", "Plots.0 6.Y-Axis", "Plots.0 7.Y-Axis", "Plots.0 8.Y-Axis", "Plots.0 9.Y-Axis", "Plots.0 10.Y-Axis", "Plots.0 11.Y-Axis", "Plots.0 12.Y-Axis", "Plots.0 13.Y-Axis", "Plots.0 14.Y-Axis", "Plots.0 15.Y-Axis", "Plots.0 16.Y-Axis", "Plots.0.Plot Color", "Plots.0 2.Plot Color", "Plots.0 3.Plot Color", "Plots.0 4.Plot Color", "Plots.0 5.Plot Color", "Plots.0 6.Plot Color", "Plots.0 7.Plot Color", "Plots.0 8.Plot Color", "Plots.0 9.Plot Color", "Plots.0 10.Plot Color", "Plots.0 11.Plot Color", "Plots.0 12.Plot Color", "Plots.0 13.Plot Color", "Plots.0 14.Plot Color", "Plots.0 15.Plot Color", "Plots.0 16.Plot Color", "Plots.0.Point Color", "Plots.0 2.Point Color", "Plots.0 3.Point Color", "Plots.0 4.Point Color", "Plots.0 5.Point Color", "Plots.0 6.Point Color", "Plots.0 7.Point Color", "Plots.0 8.Point Color", "Plots.0 9.Point Color", "Plots.0 10.Point Color", "Plots.0 11.Point Color", "Plots.0 12.Point Color", "Plots.0 13.Point Color", "Plots.0 14.Point Color", "Plots.0 15.Point Color", "Plots.0 16.Point Color": Value Change {
        w317 = refnum<vi> refnum  # ColorBox
        w328 = refnum<vi> refnum  # Ring
        w331 = refnum<vi> refnum  # Cluster
        w336 = refnum<vi> refnum  # Cluster
        n205 = event-data() -> ("CtlRef"=w335:refnum<vi>)  [unwired: 1 in]
        n206 = property class="Ctl"(reference=w335) -> (error out=w338:errorcluster, "Owner"=w337:refnum<vi>)  [unwired: 1 in, 1 out]
        n207 = To More Specific Class(target class=w336, reference=w337, error in=w338) -> (specific class reference=w333:refnum<vi>)  [unwired: 1 out]
        n208 = property class="Clust"(reference=w333) -> ("Owner"=w332:refnum<vi>, "Controls[]"=w319:refnum<vi>[])  [unwired: 1 in, 2 out]
        n209 = Index Array(array=w319, index #1=4 ("index")) -> (element #1=w322:refnum<vi>, element #2=w321:refnum<vi>, element #3=w320:refnum<vi>)  [unwired: 2 in]
        n210 = To More Specific Class(target class=w328, reference=w322) -> (specific class reference=w327:refnum<vi>)  [unwired: 1 in, 1 out]
        n211 = To More Specific Class(target class=w317, reference=w321) -> (specific class reference=w326:refnum<vi>)  [unwired: 1 in, 1 out]
        n212 = To More Specific Class(target class=w317, reference=w320) -> (specific class reference=w325:refnum<vi>)  [unwired: 1 in, 1 out]
        n213 = property class="ColBox"(reference=w326) -> ("Value"=w314:u32)  [unwired: 1 in, 2 out]
        n214 = property class="ColBox"(reference=w325) -> ("Value"=w313:u32)  [unwired: 1 in, 2 out]
        n215 = property class="Ring"(reference=w327) -> ("Value"=w324:variant)  [unwired: 1 in, 2 out]
        n216 = To More Specific Class(target class=w331, reference=w332) -> (specific class reference=w330:refnum<vi>)  [unwired: 1 in, 1 out]
        n217 = property class="Clust"(reference=w330) -> ("Controls[]"=w329:refnum<vi>[])  [unwired: 1 in, 2 out]
        n218 = Variant To Data(type=u8 0 ("unsigned 8bit integer"), Variant=w324) -> (data=w315:u8)  [unwired: 1 in, 1 out]
        n219 = Search 1D Array(1D array=w329, element=w333) -> (index of element=w334:i32)  [unwired: 1 in]
        n220 = property on="Graph" class="XYGraph (strict)"("Active Plot"=w334) -> (error out=w316:errorcluster)  [unwired: 2 in, 1 out]
        n221 = property on="Graph" class="XYGraph (strict)"(error in=w316, "Plot.Fill/Pt. Color"=w313) -> ()  [unwired: 1 in, 2 out]
        n222 = property on="Graph" class="XYGraph (strict)"(error in=w316, "Plot.YScaleIdx"=w315) -> ()  [unwired: 1 in, 2 out]
        n223 = property on="Graph" class="XYGraph (strict)"(error in=w316, "Plot.Plot Color"=w314) -> ()  [unwired: 1 in, 2 out]
      }
    }
  }
